vi "Set Grass Coupling Monitor [GPL].vi"(7 "Micropulse # In":i32, 8 "error in (no error)":errorcluster, 9 "Coupling Level":u32 caption="[GPL]" max=4095 step=1, 11 "Test Number":u32) -> (0 "error out":errorcluster, 5 "Micropulse # Out":i32)   [LabVIEW 2026, in "MicroPulse_Driver.lvlib"]
doc: "Provides facility to monitor coupling integrity using the average of amplitude of signals within the specified gated area (GAT). Generally used with high gain to enhance the ultrasonic noise of the material. The reported data indicates the total of all amplitude values in the gate (i.e. the integral of the waveform) and the average signal height. The average value is used to determine whether the data is reported, if the average is below the level specified in the GPL command a message is reported, otherwise there is no message.\n\nParameters:\n<Tn> : Test number. An integer value from 0 to the maximum number of tests (default maximum is 1279 tests).\nTn = 0 for all conventional tests. If the S extension is used it applies to all tests in the sweep number specified: 1-32, 0 = all sweeps.\n\n<Value> :\nInteger between 10 and 255 (8-bit modes)\nInteger between 10 and 1023 (10-bit modes)\nInteger between 10 and 4095 (12-bit modes)"
uses:
  MicroPulse_Driver.lvlib
  Private/MP-Registry Action-Enum.ctl
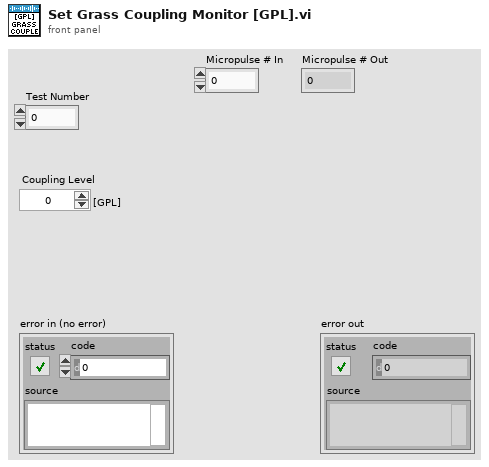
[diagram p1: front panel]
types:
  T1 = typedef "MicroPulse_Driver.lvlib/TCP config.ctl" = cluster{"Connection ID":refnum<k5>, "IP address":string, "host port":u16, "OC timeout":i32, "Read timeout":i32, "Write timeout":i32}
  T2 = typedef "MicroPulse_Driver.lvlib/MP-Registry Action-Enum.ctl" = enum16{"Read", "Add Test", "Add Command", "Add Gate Command", "Add Encoder Command", "Clear Command  List", "Set Registry", "Set System Details", "Set DOF", "Set Velocity", "Disable Asynch Reads", "Enable Asynch Reads", "Add Connection", "Disconnect", "Shutdown"}
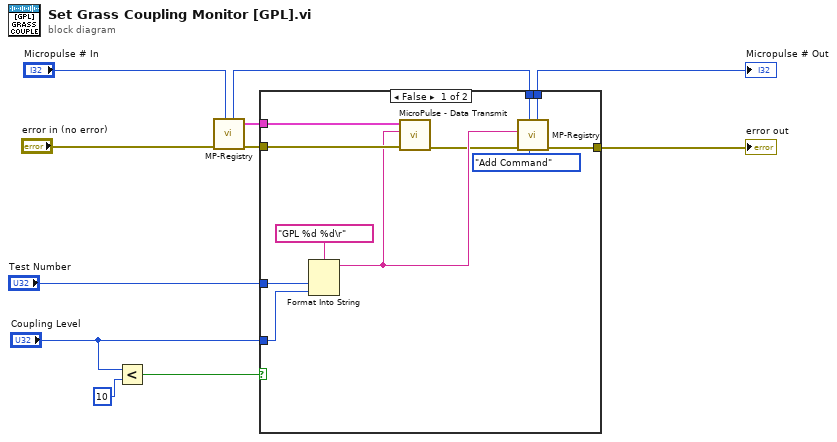
[diagram p0: block diagram]
diagram:
  n1 = Less?(x="Coupling Level", y=u32 10) -> (x < y?=w1:bool)
  n2 = call "MP-Registry.vi"("Micropulse # In"="Micropulse # In", "error in (no error)"="error in (no error)") -> ("error out"=w9:errorcluster, "TCP config"=w8:T1, "Micropulse # Out"=w5:i32)  [unwired: 6 in, 1 out]
  n3 = case shown="False" w1 {
    tunnel: w9 -> [w22 w23]
    tunnel: w8 -> [w21 _]
    tunnel: "Test Number" -> [w20 _]
    tunnel: [w16 w23] -> w6
    tunnel: w5 -> [w15 w24]
    tunnel: [w14 w24] -> w4
    tunnel: "Coupling Level" -> [w13 _]
    frame False {
      n4 = Format Into String(format string="GPL %d %d\r", w20, w13) -> (resulting string=w19:string)  [unwired: 2 in, 1 out]
      n5 = call "MicroPulse - Data Transmit.vi"("error in (no error)"=w22, "data"=w19, "TCP config"=w21) -> ("error out"=w17:errorcluster)  [unwired: 6 in, 2 out]
      n6 = call "MP-Registry.vi"("Action"=MP-Registry_Action-Enum."Add Command", "Micropulse # In"=w15, "error in (no error)"=w17, "Data in"=w19) -> ("error out"=w16:errorcluster, "Micropulse # Out"=w14:i32)  [unwired: 4 in, 2 out]
    }
    frame True {
      # "Grass coupling is turned off by issuing the AMP command"
      # "#TODO:\nRemove Grass Coupling from command list"
    }
  }
  "error out" <- w6
  "Micropulse # Out" <- w4
